vi "LL_DELETE Bucket.vi"(8 "error in (no error)":errorcluster, 9 "Bucket":string, 10 "Path and query string":string="/", 11 "Headers":T1[](array[typedef])) -> (0 "error out":errorcluster, 1 "Call Result":T2)   [LabVIEW 2011, in "LV Interface for Amazon S3.lvlib"]
doc: "This core implementation of the DELETE operation may be used to implement special requests or API calls not present in this toolkit."
uses:
  LV Interface for Amazon S3.lvlib
  Typedefs/AMZ_S3_Call Results.ctl
  Typedefs/AMZ_S3_HTTP Header-Value pair.ctl
  <vilib>/httpClient/LabVIEWHTTPClient.lvlib
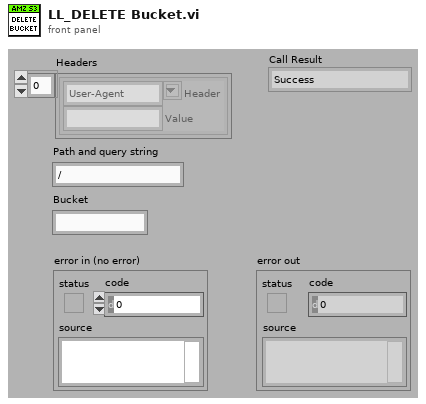
[diagram p1: front panel]
types:
  T1 = typedef "LV Interface for Amazon S3.lvlib/AMZ_S3_HTTP Header-Value pair.ctl" = cluster{"Header":string, "Value":string}
  T2 = typedef "LV Interface for Amazon S3.lvlib/AMZ_S3_Call Results.ctl" = enum16{"Success", "UndefinedError", "AccessDenied", "AccountProblem", "AmbiguousGrantByEmailAddress", "BadDigest", "BucketAlreadyExists", "BucketAlreadyOwnedByYou", "BucketNotEmpty", "CredentialsNotSupported", "CrossLocationLoggingProhibited", "EntityTooSmall", "EntityTooLarge", "ExpiredToken", "IllegalVersioningConfigurationException", "IncompleteBody", "IncorrectNumberOfFilesInPostRequest", "InlineDataTooLarge", "InternalError", "InvalidAccessKeyId", "InvalidAddressingHeader", "InvalidArgument", "InvalidBucketName", "InvalidDigest", "InvalidLocationConstraint", "InvalidPart", "InvalidPartOrder", "InvalidPayer", "InvalidPolicyDocument", "InvalidRange", "InvalidSecurity", "InvalidSOAPRequest", "InvalidStorageClass", "InvalidTargetBucketForLogging", "InvalidToken", "InvalidURI", "KeyTooLong", "MalformedACLError", "MalformedPOSTRequest", "MalformedXML", "MaxMessageLengthExceeded", "MaxPostPreDataLengthExceededError", "MetadataTooLarge", "MethodNotAllowed", "MissingAttachment", "MissingContentLength", "MissingRequestBodyError", "MissingSecurityElement", "MissingSecurityHeader", "NoLoggingStatusForKey", "NoSuchBucket", "NoSuchKey", "NoSuchUpload", "NoSuchVersion", "NotImplemented", "NotSignedUp", "OperationAborted", "PermanentRedirect", "PreconditionFailed", "Redirect", "RequestIsNotMultiPartContent", "RequestTimeout", "RequestTimeTooSkewed", "RequestTorrentOfBucketError", "SignatureDoesNotMatch", "SlowDown", "TemporaryRedirect", "TokenRefreshRequired", "TooManyBuckets", "UnexpectedContent", "UnresolvableGrantByEmailAddress", "UserKeyMustBeSpecified", "LabVIEWError"}
  T3 = typedef "LabVIEWHTTPClient.lvlib/ClientHandle.ctl" = refnum<k1>
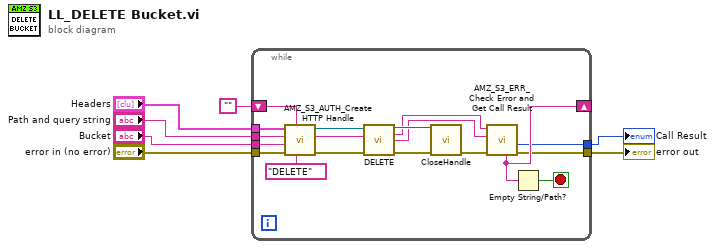
[diagram p0: block diagram]
diagram:
  n1 = while {
    tunnel: "error in (no error)" -> [w24]
    tunnel: "Bucket" -> [w23]
    tunnel: "Path and query string" -> [w22]
    tunnel: "Headers" -> [w21]
    shift-right: [w10] -> _
    shift-left: "" -> [w20]
    tunnel: [w9] -> w6
    tunnel: [w8] -> w5
    stop <- w11 stop-if-true
    n2 = call "AMZ_S3_AUTH_Create HTTP Handle.vi"("HTTP-Verb"="DELETE", "Redirect endpoint"=w20, "error in (no error)"=w24, "Bucket"=w23, "Path and query string"=w22, "Headers"=w21) -> ("error out"=w19:errorcluster, "URL"=w18:string, "client handle out"=w17:T3)  [unwired: 3 in]
    n3 = call <vilib>:"DELETE.vi"("client handle"=w17, "url"=w18, "error in (no error)"=w19) -> ("client handle out"=w16:T3, "headers"=w13:string, "body"=w12:string, "error out"=w15:errorcluster)  [unwired: 9 in]
    n4 = call <vilib>:"CloseHandle.vi"("client handle"=w16, "error in (no error)"=w15) -> ("error out"=w14:errorcluster)  [unwired: 13 in]
    n5 = call "AMZ_S3_ERR_Check Error and Get Call Result.vi"("error in (no error)"=w14, "Response body"=w12, "Response header"=w13) -> ("error out"=w9:errorcluster, "Call Result"=w8:T2, "Redirect endpoint"=w10:string)  [unwired: 4 in, 2 out]
    n6 = Empty String/Path?(string/path=w10) -> (empty?=w11:bool)
  }
  "error out" <- w6
  "Call Result" <- w5
